vi "SDCP SMF Transmitter and Receiver - Live Plot - Logger Loop.vi"(3 "error in (no error)":errorcluster, 4 "Trace File Path in":path, 5 "log queue":refnum<queue>) -> (0 "error out":errorcluster, 1 "Trace File Path out":path)   [LabVIEW 2020]
uses:
  <vilib>/Utility/file.llb/Write Delimited Spreadsheet (string).vi
  Global Stop.vi
panel:
  out "# elements in queue":i32
  out "size(s)":i32
  out "save interval (ms)":u32
  out "Save to file":bool
  out "Log data":cluster{"Record":string[]}[](array[cluster])
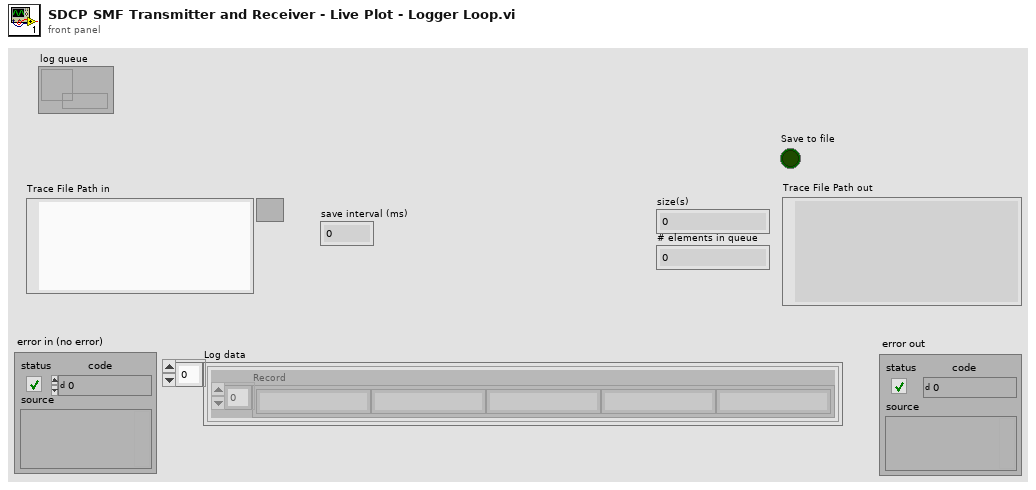
[diagram p1: front panel]
types:
  T1 = enum16{"open", "replace", "create", "open or create", "replace or create", "replace or create with confirmation"}
  T2 = cluster{"data bytes":u8[], "Time (ms)":u32, "Direction":string}
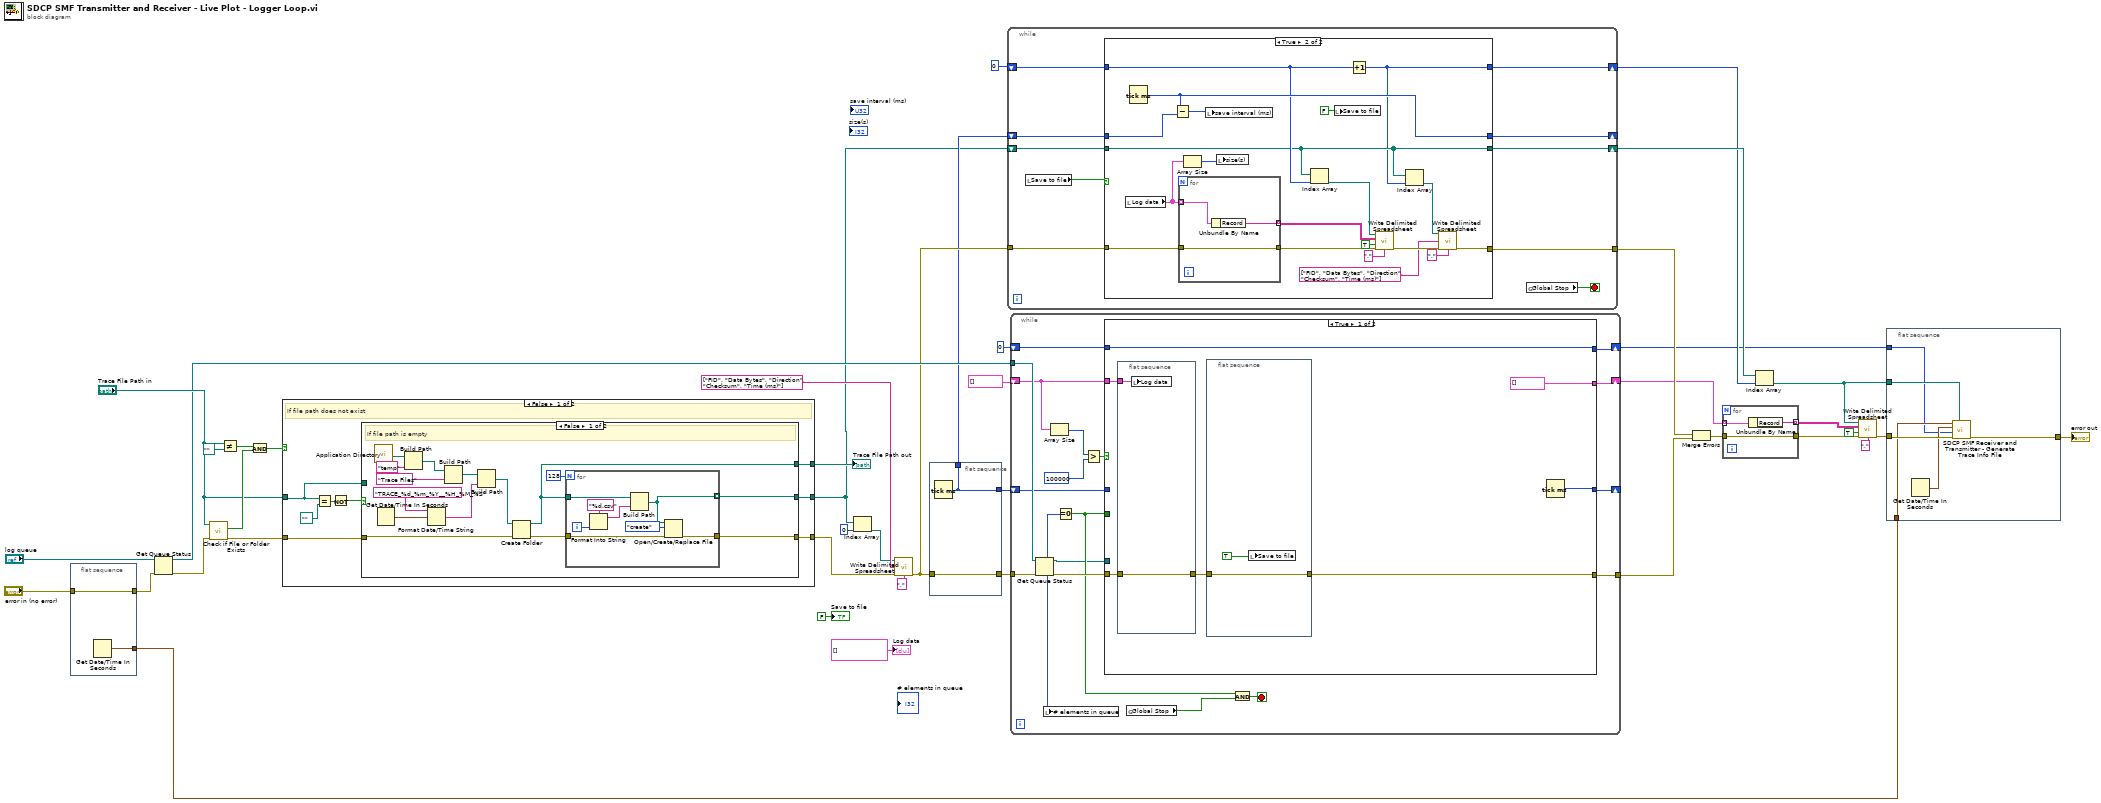
[diagram p0: block diagram]
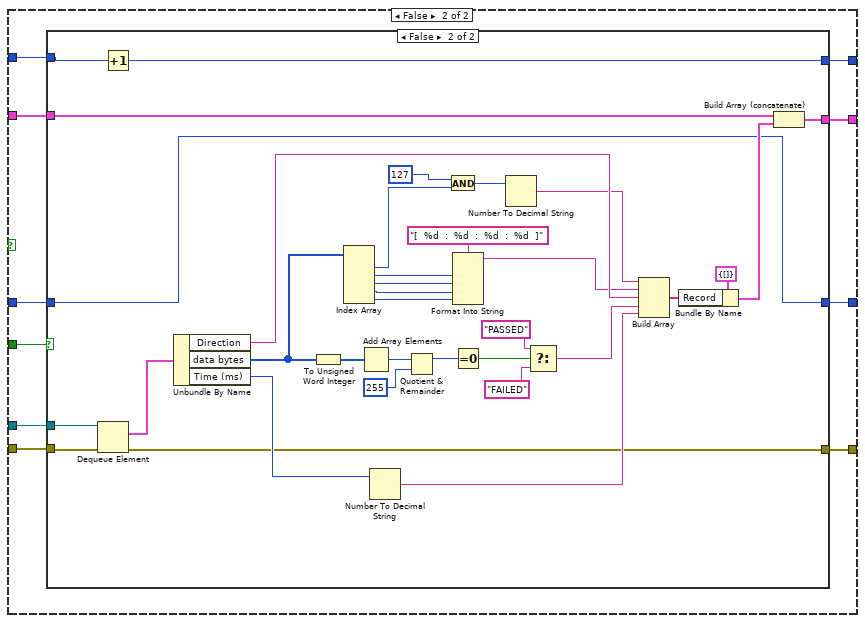
[diagram p3: hidden frame]
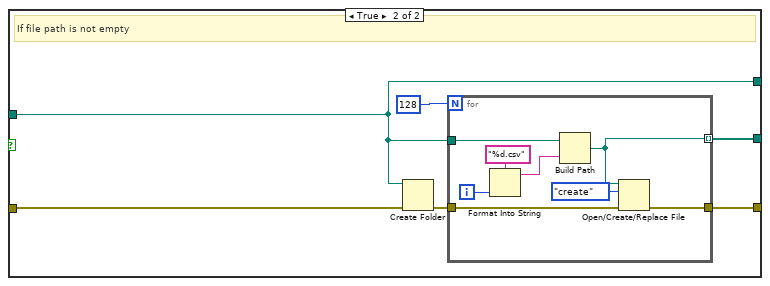
[diagram p5: hidden frame]
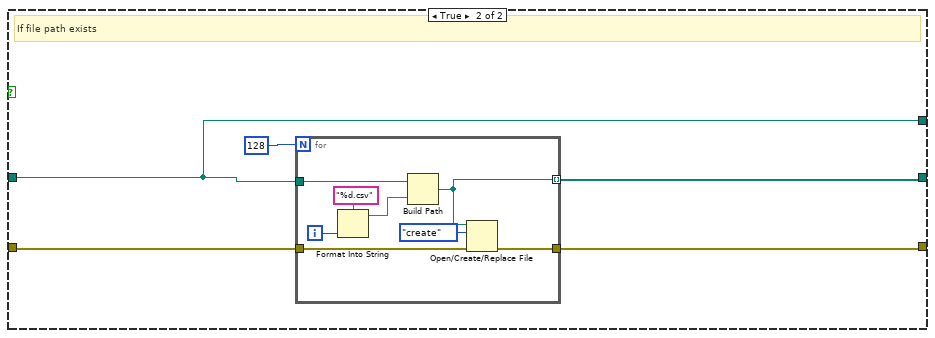
[diagram p6: hidden frame]
diagram:
  n1 = flat-sequence {
    tunnel: "error in (no error)" -> [w44]
    tunnel: [w44] -> w7
    tunnel: [w43] -> w3
    frame #0 {
      n2 = Get Date/Time In Seconds() -> (seconds since 1Jan1904=w43:timestamp)
    }
  }
  n3 = Get Queue Status(queue="log queue", error in (no error)=w7) -> (queue out=w31:refnum<queue>, error out=w33:errorcluster)  [unwired: 1 in, 6 out]
  n4 = call <vilib>:"Check if File or Folder Exists.vi"("error in (no error)"=w33, "path"="Trace File Path in") -> ("error out"=w41:errorcluster, "file or folder exists?"=w36:bool)  [unwired: 7 in, 1 out]
  n5 = Not Equal?(x="Trace File Path in", y=path "") -> (x != y?=w35:bool)
  n6 = And(x=w35, y=w36) -> (x .and. y?=w37:bool)
  n7 = case shown="False" w37 {
    tunnel: w41 -> [w52 w92]
    tunnel: "Trace File Path in" -> [w50 w90]
    tunnel: [w51 w91] -> w40
    tunnel: [w46 w93] -> w20
    tunnel: [w45 w90] -> w21
    frame False {
      # "If file path does not exist"
      n8 = Equal?(x=w50, y=path "") -> (x = y?=w48:bool)
      n9 = Not(x=w48) -> (.not. x?=w47:bool)
      n10 = case shown="False" w47 {
        tunnel: w52 -> [w59 w81]
        tunnel: w50 -> [_ w76]
        tunnel: [w55 w78] -> w51
        tunnel: [w56 w77] -> w46
        tunnel: [w54 w76] -> w45
        frame False {
          # "If file path is empty"
          n11 = call <vilib>:"Application Directory.vi"() -> ("Application Directory"=w67:path)
          n12 = Get Date/Time In Seconds() -> (seconds since 1Jan1904=w62:timestamp)
          n13 = Build Path(base path=w67, name or relative path="temp") -> (appended path=w65:path)
          n14 = Format Date/Time String(time format string (%c)="TRACE_%d_%m_%Y__%H_%M_%S", seconds (now)=w62) -> (date/time string=w60:string)  [unwired: 1 in]
          n15 = Build Path(base path=w65, name or relative path="Trace Files") -> (appended path=w63:path)
          n16 = Build Path(base path=w63, name or relative path=w60) -> (appended path=w58:path)
          n17 = Create Folder(path (use dialog)=w58, error in=w59) -> (created path=w54:path, error out=w57:errorcluster)  [unwired: 1 in, 1 out]
          n18 = for {
            N: 128 -> [_]
            tunnel: w54 -> [w75]
            tunnel: w57 -> [w71]
            tunnel: [w69] -> w55
            tunnel: [w68] -> w56 mode=indexing
            i -> [w73]
            n19 = Format Into String(format string="%d.csv", w73) -> (resulting string=w72:string)  [unwired: 2 in, 1 out]
            n20 = Build Path(base path=w75, name or relative path=w72) -> (appended path=w68:path)
            n21 = Open/Create/Replace File(file path (use dialog)=w68, error in=w71, operation (0:open)=T1."create") -> (error out=w69:errorcluster)  [unwired: 3 in, 2 out]
          }
        }
        frame True {
          # "If file path is not empty"
          n22 = Create Folder(path (use dialog)=w76, error in=w81) -> (error out=w80:errorcluster)  [unwired: 1 in, 2 out]
          n23 = for {
            N: 128 -> [_]
            tunnel: w76 -> [w89]
            tunnel: w80 -> [w85]
            tunnel: [w83] -> w78
            tunnel: [w82] -> w77 mode=indexing
            i -> [w87]
            n24 = Format Into String(format string="%d.csv", w87) -> (resulting string=w86:string)  [unwired: 2 in, 1 out]
            n25 = Build Path(base path=w89, name or relative path=w86) -> (appended path=w82:path)
            n26 = Open/Create/Replace File(file path (use dialog)=w82, error in=w85, operation (0:open)=T1."create") -> (error out=w83:errorcluster)  [unwired: 3 in, 2 out]
          }
        }
      }
    }
    frame True {
      # "If file path exists"
      n27 = for {
        N: 128 -> [_]
        tunnel: w90 -> [w102]
        tunnel: w92 -> [w98]
        tunnel: [w96] -> w91
        tunnel: [w95] -> w93 mode=indexing
        i -> [w100]
        n28 = Format Into String(format string="%d.csv", w100) -> (resulting string=w99:string)  [unwired: 2 in, 1 out]
        n29 = Build Path(base path=w102, name or relative path=w99) -> (appended path=w95:path)
        n30 = Open/Create/Replace File(file path (use dialog)=w95, error in=w98, operation (0:open)=T1."create") -> (error out=w96:errorcluster)  [unwired: 3 in, 2 out]
      }
    }
  }
  "Trace File Path out" <- w21
  n31 = Index Array(array=w20, index=0) -> (element=w19:path)
  n32 = call-poly <vilib>:"Write Delimited Spreadsheet.vi"("file path (dialog if empty)"=w19, "1D data"=string[] ["FID", "Data Bytes", "Direction", "Checksum", "Time (ms)"], "error in (no error)"=w40, "delimiter (\\t)"="," ("delimiter (\\t)")) -> ("error out"=w27:errorcluster)  [unwired: 10 in, 1 out]
  n33 = flat-sequence {
    tunnel: w27 -> [w104]
    tunnel: [w104] -> w30
    tunnel: [w103] -> w29
    tunnel: [w103] -> w26
    frame #0 {
      n34 = Tick Count (ms)() -> (millisecond timer value=w103:u32)
    }
  }
  n35 = while {
    tunnel: w27 -> [w113]
    shift-right: [w109] -> _
    shift-left: w26 -> [w110]
    tunnel: [w111] -> w24
    shift-right: [w107] -> w16
    shift-left: w20 -> [w112]
    shift-right: [w105] -> w9
    shift-left: 0 -> [w106]
    stop <- w108 stop-if-true
    n36 = local read "Save to file"() -> (w114:bool)
    n37 = case shown="True" w114 {
      tunnel: w113 -> [w117 w138]
      tunnel: w112 -> [w116 w123]
      tunnel: [w117 w120] -> w111
      tunnel: w110 -> [w118 w134]
      tunnel: [w118 w133] -> w109
      tunnel: [w116 w123] -> w107
      tunnel: w106 -> [w115 w128]
      tunnel: [w115 w122] -> w105
      frame False {
      }
      frame True {
        n38 = local read "Log data"() -> (w131:cluster{"Record":string[]}[])
        n39 = Tick Count (ms)() -> (millisecond timer value=w133:u32)
        n40 = Subtract(x=w133, y=w134) -> (x-y=w130:u32)
        n41 = for {
          tunnel: w138 -> [w139]
          tunnel: w131 -> [w141] mode=indexing
          tunnel: [w140] -> w126 mode=indexing
          tunnel: [w139] -> w137
          n42 = Unbundle By Name(w141) -> ("Record"=w140:string[])
        }
        n43 = Array Size(array=w131) -> (size(s)=w129:i32)
        n44 = local write "save interval (ms)"(w130) -> ()
        n45 = local write "size(s)"(w129) -> ()
        n46 = Index Array(array=w123, index=w128) -> (element=w127:path)
        n47 = local write "Save to file"(FALSE ("Save to file")) -> ()
        n48 = Increment(x=w128) -> (x+1=w122:i32)
        n49 = call-poly <vilib>:"Write Delimited Spreadsheet.vi"("file path (dialog if empty)"=w127, "2D data"=w126, "append to file? (new file:F)"=TRUE, "error in (no error)"=w137, "delimiter (\\t)"="," ("delimiter (\\t)")) -> ("error out"=w125:errorcluster)  [unwired: 9 in, 1 out]
        n50 = Index Array(array=w123, index=w122) -> (element=w121:path)
        n51 = call-poly <vilib>:"Write Delimited Spreadsheet.vi"("file path (dialog if empty)"=w121, "1D data"=string[] ["FID", "Data Bytes", "Direction", "Checksum", "Time (ms)"], "error in (no error)"=w125, "delimiter (\\t)"="," ("delimiter (\\t)")) -> ("error out"=w120:errorcluster)  [unwired: 10 in, 1 out]
      }
    }
    n52 = global read "Global Stop.vi" "Global Stop"() -> (w108:bool)
  }
  n53 = while {
    tunnel: w30 -> [w159]
    tunnel: w31 -> [w158]
    shift-right: [w149] -> _
    shift-left: w29 -> [w150]
    shift-right: [w152] -> w12
    shift-left: cluster{"Record":string[]}[] [] -> [w147]
    tunnel: [w151] -> w25
    shift-right: [w142] -> w1
    shift-left: u32 0 -> [w143]
    stop <- w156 stop-if-true
    n54 = Get Queue Status(queue=w158, error in (no error)=w159) -> (queue out=w153:refnum<queue>, error out=w157:errorcluster, # elements in queue=w148:i32)  [unwired: 1 in, 5 out]
    n55 = local write "# elements in queue"(w148) -> ()
    n56 = Array Size(array=w147) -> (size(s)=w145:i32)
    n57 = Equal To 0?(x=w148) -> (x = 0?=w155:bool)
    n58 = Greater?(x=w145, y=100000) -> (0:w146:bool)
    n59 = case shown="True" w146 {
      tunnel: w157 -> [w163 w180]
      tunnel: w155 -> [_ w179]
      tunnel: w153 -> [_ w178]
      tunnel: w147 -> [w164 w177]
      tunnel: [cluster{"Record":string[]}[] [] w176] -> w152
      tunnel: [w161 w175] -> w151
      tunnel: w150 -> [_ w174]
      tunnel: [w165 w173] -> w149
      tunnel: w143 -> [w160 w172]
      tunnel: [w160 w171] -> w142
      frame True {
        n60 = flat-sequence {
          tunnel: w164 -> [w170]
          tunnel: w163 -> [w169]
          tunnel: [w169] -> w162
          frame #0 {
            n61 = local write "Log data"(w170) -> ()
          }
        }
        n62 = flat-sequence {
          tunnel: w162 -> [w167]
          tunnel: [w167] -> w161
          frame #0 {
            n63 = local write "Save to file"(TRUE ("Save to file")) -> ()
          }
        }
        n64 = Tick Count (ms)() -> (millisecond timer value=w165:u32)
      }
      frame False {
        n65 = case shown="False" w179 {
          tunnel: w180 -> [w183 w194]
          tunnel: w178 -> [_ w193]
          tunnel: w177 -> [w184 w191]
          tunnel: [w184 w189] -> w176
          tunnel: [w183 w188] -> w175
          tunnel: w174 -> [w182 w187]
          tunnel: [w182 w187] -> w173
          tunnel: w172 -> [w181 w186]
          tunnel: [w181 w185] -> w171
          frame True {
          }
          frame False {
            n66 = Dequeue Element(queue=w193, error in (no error)=w194) -> (element=w192:T2, error out=w188:errorcluster)  [unwired: 1 in, 2 out]
            n67 = Increment(x=w186) -> (x+1=w185:u32)
            n68 = Unbundle By Name(w192) -> ("Direction"=w202:string, "data bytes"=w213:u8[], "Time (ms)"=w203:u32)
            n69 = To Unsigned Word Integer(number=w213) -> (unsigned 16bit integer=w212:u16[])
            n70 = Index Array(array=w213) -> (element #1=w200:u8, element #2=w217:u8, element #3=w216:u8, element #4=w215:u8, element #5=w214:u8)  [unwired: 5 in]
            n71 = Add Array Elements(numeric array=w212) -> (sum=w211:u16)
            n72 = Number To Decimal String(number=w203) -> (decimal integer string=w205:string)  [unwired: 1 in]
            n73 = Quotient & Remainder(x=w211, y=u16 255) -> (x-y*floor(x/y)=w209:u16)  [unwired: 1 out]
            n74 = And(x=u8 127, y=w200) -> (x .and. y?=w198:u8)
            n75 = Format Into String(format string="[  %d  :  %d  :  %d  :  %d  ]", w217, w216, w215, w214) -> (resulting string=w201:string)  [unwired: 2 in, 1 out]
            n76 = Equal To 0?(x=w209) -> (x = 0?=w208:bool)
            n77 = Number To Decimal String(number=w198) -> (decimal integer string=w197:string)  [unwired: 1 in]
            n78 = Select(t="PASSED", s=w208, f="FAILED") -> (s? t:f=w204:string)
            n79 = Build Array(w197, w201, w202, w204, w205) -> (w195:string[])
            n80 = Bundle By Name(cluster=cluster{"Record":string[]} {"Record"=[]}, "Record"=w195) -> (w190:cluster{"Record":string[]})
            n81 = Build Array (concatenate)(w191, w190) -> (w189:cluster{"Record":string[]}[])
          }
        }
      }
    }
    n82 = global read "Global Stop.vi" "Global Stop"() -> (w154:bool)
    n83 = And(x=w155, y=w154) -> (x .and. y?=w156:bool)
  }
  n84 = Merge Errors(w24, w25) -> (w14:errorcluster)
  n85 = for {
    tunnel: w14 -> [w221]
    tunnel: [w221] -> w13
    tunnel: w12 -> [w220] mode=indexing
    tunnel: [w219] -> w11 mode=indexing
    n86 = Unbundle By Name(w220) -> ("Record"=w219:string[])
  }
  n87 = Index Array(array=w16, index=w9) -> (element=w4:path)
  n88 = call-poly <vilib>:"Write Delimited Spreadsheet.vi"("file path (dialog if empty)"=w4, "2D data"=w11, "append to file? (new file:F)"=TRUE, "error in (no error)"=w13, "delimiter (\\t)"="," ("delimiter (\\t)")) -> ("error out"=w6:errorcluster)  [unwired: 9 in, 1 out]
  n89 = flat-sequence {
    tunnel: w6 -> [w227]
    tunnel: [w226] -> w5
    tunnel: w4 -> [w225]
    tunnel: w3 -> [w223]
    tunnel: w1 -> [w222]
    frame #0 {
      n90 = Get Date/Time In Seconds() -> (seconds since 1Jan1904=w224:timestamp)
      n91 = call "SDCP SMF Receiver and Transmitter - Generate Trace Info File.vi"("Trace File Path"=w225, "error in (no error)"=w227, "Number of samples"=w222, "Stop Time"=w224, "Start Time"=w223) -> ("error out"=w226:errorcluster)  [unwired: 6 in]
    }
  }
  "error out" <- w5
  "Save to file" <- FALSE ("Save to file")
  "Log data" <- cluster{"Record":string[]}[] [] ("Log data")
